vi "Move Motor.vi"(6 "Goal Speed (RPM)":dbl, 8 "error in (no error)":errorcluster, 9 "Goal Position (150 deg)":dbl=150.0, 10 "Motor ID (0)":u8, 11 "Dynamixel Motor VISA in":refnum<class "Dynamixel Motor VISA.lvclass">) -> (0 "error out":errorcluster, 3 "Dynamixel Motor VISA out":refnum<class "Dynamixel Motor VISA.lvclass">)   [LabVIEW 2016, in "Dynamixel Motor VISA.lvclass"]
doc: "Sets the goal position for the motor."
uses:
  <instrlib>/Dynamixel Motor/HAIOL/VISA/Dynamixel Motor VISA.lvclass
  <instrlib>/Dynamixel Motor/HAIOL/VISA/Dynamixel Motor VISA.lvclass/Dynamixel Motor VISA.ctl
  <instrlib>/Dynamixel Motor/Dynamixel Motor.lvlib
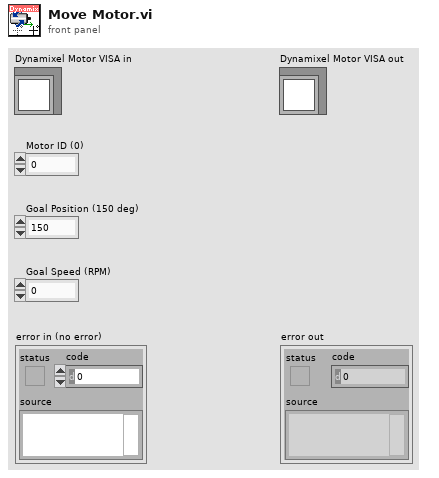
[diagram p1: front panel]
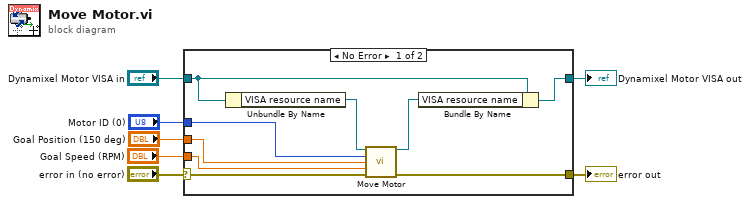
[diagram p0: block diagram]
diagram:
  n1 = case shown="No Error" "error in (no error)" {
    selector: "error in (no error)" -> [w16 w17]
    tunnel: "Dynamixel Motor VISA in" -> [w10 w18]
    tunnel: "Motor ID (0)" -> [w14 _]
    tunnel: "Goal Position (150 deg)" -> [w13 _]
    tunnel: "Goal Speed (RPM)" -> [w12 _]
    tunnel: [w11 w17] -> w2
    tunnel: [w8 w18] -> w1
    frame No Error {
      n2 = Unbundle By Name(w10) -> ("VISA resource name"=w15:refnum<visa-resource-name>)
      n3 = call <instrlib>:"Move Motor.vi"("VISA resource name"=w15, "Motor ID (0)"=w14, "Goal Position (150 deg)"=w13, "Goal Speed (RPM)"=w12, "error in (no error)"=w16) -> ("VISA resource name out"=w9:refnum<visa-resource-name>, "error out"=w11:errorcluster)  [unwired: 9 in]
      n4 = Bundle By Name(cluster=w10, "VISA resource name"=w9) -> (w8:refnum<class "Dynamixel Motor VISA.lvclass">)
    }
    frame Error {
    }
  }
  "error out" <- w2
  "Dynamixel Motor VISA out" <- w1
